vi "Filenames 3d.vi"(10 "Z Slice":i16, 11 "Filenames In":string[](array[string])) -> (3 "Filenames Out":string[](array[string]))   [LabVIEW 2023]
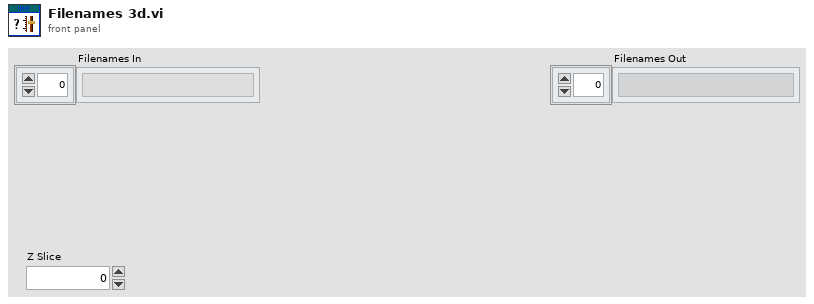
[diagram p1: front panel]
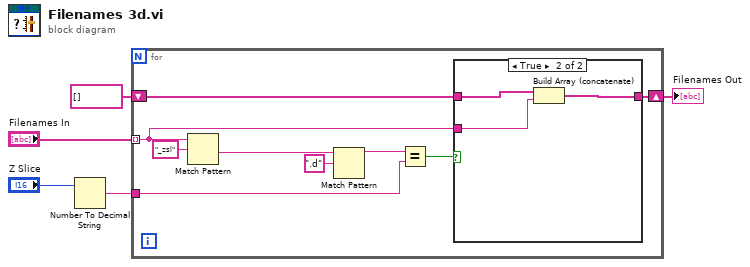
[diagram p0: block diagram]
diagram:
  n1 = Number To Decimal String(number="Z Slice") -> (decimal integer string=w3:string)  [unwired: 1 in]
  n2 = for {
    tunnel: "Filenames In" -> [w8] mode=indexing
    tunnel: w3 -> [w10]
    shift-right: [w7] -> w1
    shift-left: string[] [] -> [w6]
    n3 = Match Pattern(string=w8, regular expression="_zsl") -> (after substring=w13:string)  [unwired: 1 in, 3 out]
    n4 = Match Pattern(string=w13, regular expression=".d") -> (before substring=w11:string)  [unwired: 1 in, 3 out]
    n5 = Equal?(x=w11, y=w10) -> (x = y?=w9:bool)
    n6 = case shown="True" w9 {
      tunnel: w8 -> [_ w18]
      tunnel: [w15 w17] -> w7
      tunnel: w6 -> [w15 w16]
      frame False {
      }
      frame True {
        n7 = Build Array (concatenate)(w16, w18) -> (w17:string[])
      }
    }
  }
  "Filenames Out" <- w1
